vi "test-COM.vi"() -> ()   [LabVIEW 2014]
uses:
  <vilib>/Instr/_visa.llb/VISA Find Search Mode.ctl
panel:
  in  "Search Mode":T1 items=["仅允许规范名称"=0, "只允许别名"=2, "包含匹配别名"=3, "包含所有别名"=4]
  out "返回数":u32
  out "查找列表":string[](array[string])
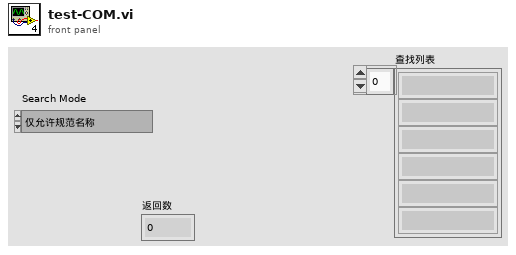
[diagram p1: front panel]
types:
  T1 = typedef "VISA Find Search Mode.ctl" = u32
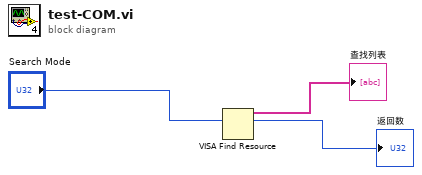
[diagram p0: block diagram]
diagram:
  n1 = VISA Find Resource(10:"Search Mode") -> (2:→"返回数":u32, 3:→"查找列表":string[])  [unwired: 2 in, 1 out]
